vi "State_Machine.vi"(8 "error in (no error)":errorcluster caption="entrée d'erreur (pas d'erreur)", 11 "Get_Voltage en entrée":refnum<class "Print_Label.lvclass">) -> (0 "error out":errorcluster caption="sortie d'erreur", 2 "Json_String":string, 3 "Get_Voltage en sortie":refnum<class "Print_Label.lvclass">)   [LabVIEW 2020, in "Library Test.lvlib" / "Print_Label.lvclass"]
uses:
  Print_Label.lvclass
  C:/Users/ngarcin/OneDrive - Altyor/Standard TB/Suite TB45/Class/Test/Test (Default)/Test (Default).lvclass
  Commun VI/TypeDef/Variable Printable.ctl
  Instrument/Instrument (Default)/Class Instrument (Default).lvclass
  Commun VI/Library Commun.lvlib
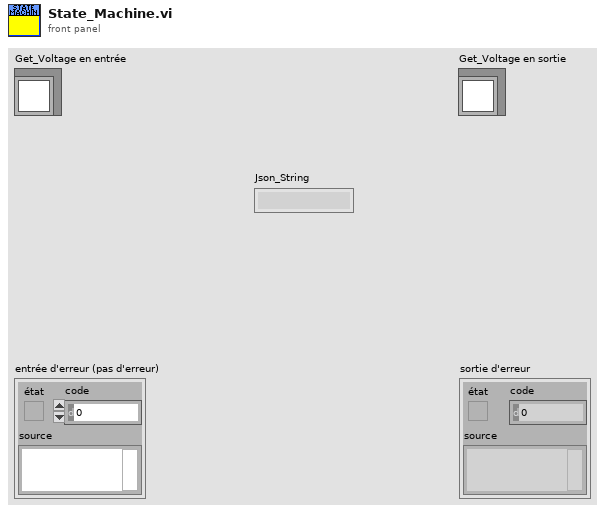
[diagram p1: front panel]
types:
  T1 = typedef "Variable Printable.ctl" = string
  T2 = enum16{"Get Variable", "Get All Variables", "Set Variable", "Delete Variable", "Delete All Variable"}
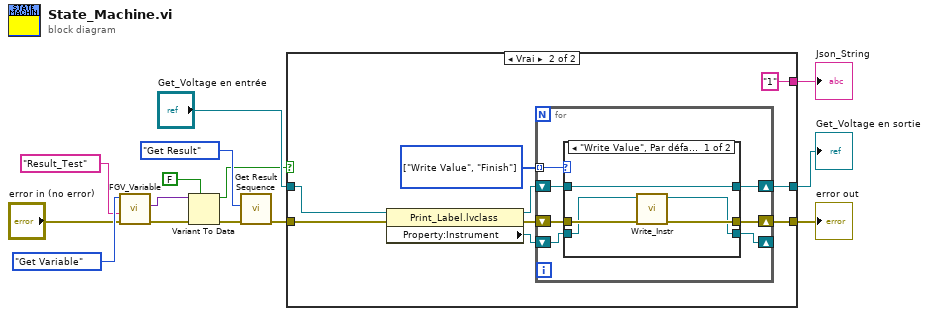
[diagram p0: block diagram]
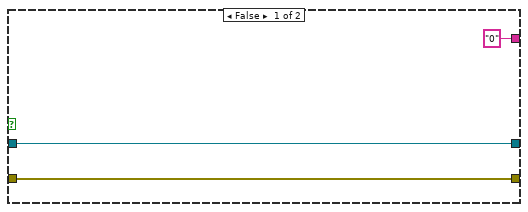
[diagram p2: hidden frame]
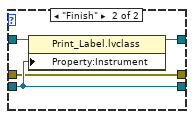
[diagram p3: hidden frame]
diagram:
  n1 = call "FGV_Variable.vi"("error in (no error)"="error in (no error)", "Variable"=T1 "Result_Test", "Function"=T2."Get Variable") -> ("error out"=w6:errorcluster, "Data Out"=w5:variant)  [unwired: 6 in, 1 out]
  n2 = Variant To Data(error in=w6, type=FALSE, Variant=w5) -> (data=w1:bool, error out=w2:errorcluster)
  n3 = call "Get Result Sequence.vi"("error in (no error)"=w2, "Function"=enum16{"Get Result", "Reset", "Set Result"}."Get Result") -> ("error out"=w11:errorcluster)  [unwired: 8 in, 1 out]
  n4 = case shown="Vrai" w1 {
    tunnel: "Get_Voltage en entrée" -> [w17 w26]
    tunnel: [w16 w22] -> w13
    tunnel: [w17 w21] -> w12
    tunnel: w11 -> [w16 w19]
    tunnel: ["0" "1"] -> w9
    frame False {
    }
    frame True {
      w25 = enum16{"Init", "Write Value", "Finish"}[] [enum."Write Value", enum."Finish"] items=["Init", "Write Value", "Finish"]
      n5 = property class="Print_Label.lvclass"(reference=w26, error in=w19) -> (reference out=w23:refnum<class "Print_Label.lvclass">, error out=w20:errorcluster, "Property:Instrument"=w24:refnum<class "Class Instrument (Default).lvclass">)
      n6 = for {
        tunnel: w25 -> [w33] mode=indexing
        shift-right: [w31] -> _
        shift-left: w24 -> [w32]
        shift-right: [w29] -> w21
        shift-left: w23 -> [w30]
        shift-right: [w27] -> w22
        shift-left: w20 -> [w28]
        n7 = case shown="\"Write Value\", Par défaut" w33 {
          tunnel: w32 -> [w34 w40]
          tunnel: [w35 w40] -> w31
          tunnel: w30 -> [w38 w42]
          tunnel: [w38 w41] -> w29
          tunnel: w28 -> [w37 w39]
          tunnel: [w36 w39] -> w27
          frame "Write Value", Default {
            n8 = call-dynamic "Write_Instr.vi"("error in (no error)"=w37, "Class Multimeter (Default) en entrée"=w34) -> ("error out"=w36:errorcluster, "Class Multimeter (Default) en sortie"=w35:refnum<class "Class Instrument (Default).lvclass">)  [unwired: 8 in]
          }
          frame "Finish" {
            n9 = property class="Print_Label.lvclass"(reference=w42, "Property:Instrument"=w40) -> (reference out=w41:refnum<class "Print_Label.lvclass">)  [unwired: 1 in, 1 out]
          }
        }
      }
    }
  }
  "error out" <- w13
  "Get_Voltage en sortie" <- w12
  "Json_String" <- w9
